vi "Update_Host.vi"(6 "Display Cluster":T1, 7 "ChangeonFly":T2, 8 "SettingsCluster":T3={"Sample Rate (us)"=1, "Samples Per Data Point (int, power of 2)"=1000, "DistanceToBulk (um)"=-1.0, "HoldTimeScaler"=1, "SaveData"=FALSE, "DistanceToBulk (um) 2"=-1.0, "DistanceToBulk (um) 3"=-1.0}, 9 "WayPointCluster":T4) -> ()   [LabVIEW 2023]
uses:
  TypeDefs/WayPointCluster.ctl
  TypeDefs/Settings.ctl
  TypeDefs/ChangeOnFly.ctl
  TypeDefs/Display.ctl
  User_Vi/Settings.vi
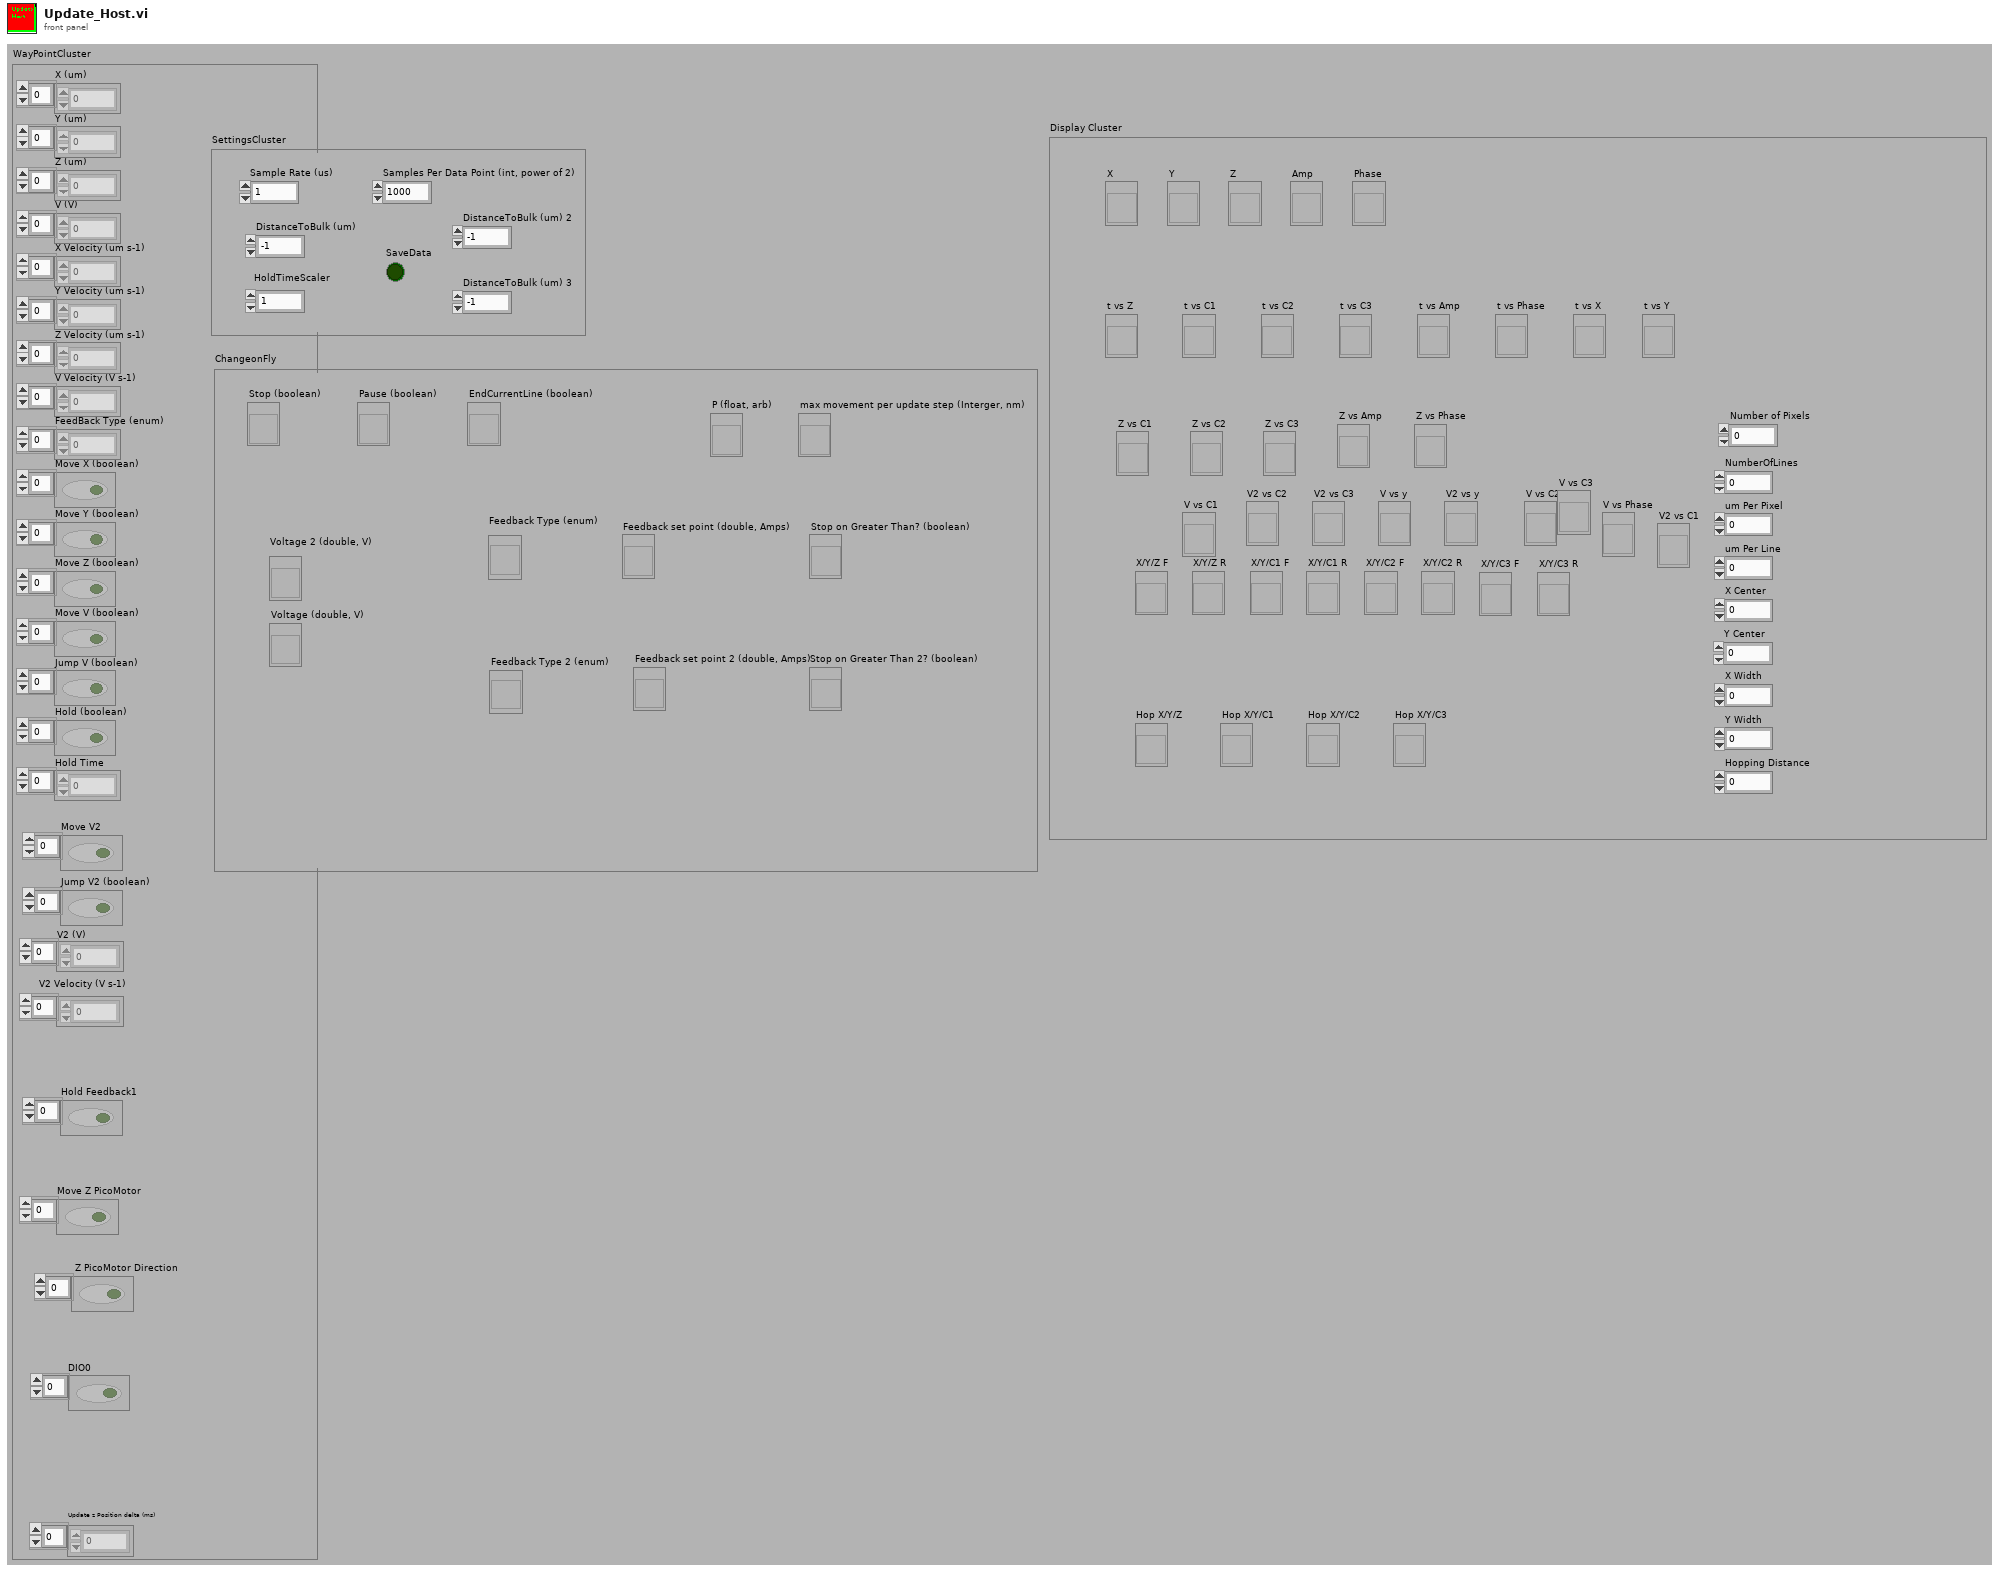
[diagram p1: front panel]
types:
  T1 = typedef "Display.ctl" = cluster{"X":refnum<vi>, "Y":refnum<vi>, "Z":refnum<vi>, "Amp":refnum<vi>, "Phase":refnum<vi>, "t vs Z":refnum<vi>, "t vs C1":refnum<vi>, "t vs C2":refnum<vi>, "t vs C3":refnum<vi>, "t vs Amp":refnum<vi>, "t vs Phase":refnum<vi>, "t vs X":refnum<vi>, "t vs Y":refnum<vi>, "Z vs C1":refnum<vi>, "Z vs C2":refnum<vi>, "Z vs C3":refnum<vi>, "V vs C1":refnum<vi>, "V vs C2":refnum<vi>, "V vs C3":refnum<vi>, "X/Y/Z F":refnum<vi>, "X/Y/Z R":refnum<vi>, "X/Y/C1 F":refnum<vi>, "X/Y/C1 R":refnum<vi>, "X/Y/C2 F":refnum<vi>, "X/Y/C2 R":refnum<vi>, "X/Y/C3 F":refnum<vi>, "X/Y/C3 R":refnum<vi>, "NumberOfLines":u16, "um Per Pixel":dbl, "um Per Line":dbl, "X Center":dbl, "Hop X/Y/Z":refnum<vi>, "Hop X/Y/C1":refnum<vi>, "Hop X/Y/C2":refnum<vi>, "Hop X/Y/C3":refnum<vi>, "X Width":dbl, "Y Width":dbl, "Hopping Distance":dbl, "V2 vs C1":refnum<vi>, "V vs Phase":refnum<vi>, "Y Center":dbl, "Number of Pixels":dbl, "V2 vs C2":refnum<vi>, "V2 vs C3":refnum<vi>, "V vs y":refnum<vi>, "V2 vs y":refnum<vi>, "Z vs Amp":refnum<vi>, "Z vs Phase":refnum<vi>}
  T2 = typedef "ChangeOnFly.ctl" = cluster{"Stop (boolean)":refnum<vi>, "Pause (boolean)":refnum<vi>, "EndCurrentLine (boolean)":refnum<vi>, "max movement per update step (Interger, nm)":refnum<vi>, "P (float, arb)":refnum<vi>, "Feedback set point (double, Amps)":refnum<vi>, "Voltage (double, V)":refnum<vi>, "Feedback set point 2 (double, Amps)":refnum<vi>, "Stop on Greater Than 2? (boolean)":refnum<vi>, "Stop on Greater Than? (boolean)":refnum<vi>, "Voltage 2 (double, V)":refnum<vi>, "Feedback Type (enum)":refnum<vi>, "Feedback Type 2 (enum)":refnum<vi>}
  T3 = typedef "Settings.ctl" = cluster{"Sample Rate (us)":u32, "Samples Per Data Point (int, power of 2)":i16, "DistanceToBulk (um)":dbl, "HoldTimeScaler":u64, "SaveData":bool, "DistanceToBulk (um) 2":dbl, "DistanceToBulk (um) 3":dbl}
  T4 = typedef "WayPointCluster.ctl" = cluster{"X (um)":dbl[], "Y (um)":dbl[], "Z (um)":dbl[], "V (V)":dbl[], "X Velocity (um s-1)":dbl[], "Y Velocity (um s-1)":dbl[], "Z Velocity (um s-1)":dbl[], "V Velocity (V s-1)":dbl[], "FeedBack Type (enum)":u16[], "Move X (boolean)":bool[], "Move Y (boolean)":bool[], "Move Z (boolean)":bool[], "Move V (boolean)":bool[], "Jump V (boolean)":bool[], "Hold (boolean)":bool[], "Hold Time":u32[], "V2 (V)":dbl[], "Move V2":bool[], "V2 Velocity (V s-1)":dbl[], "Jump V2 (boolean)":bool[], "Update z Position delta (ms)":i16[], "Hold Feedback1":bool[], "Move Z PicoMotor":bool[], " Z PicoMotor Direction":bool[], "DIO0":bool[]}
  T5 = enum32{"Bad", "Idle", "Run top level", "Running"}
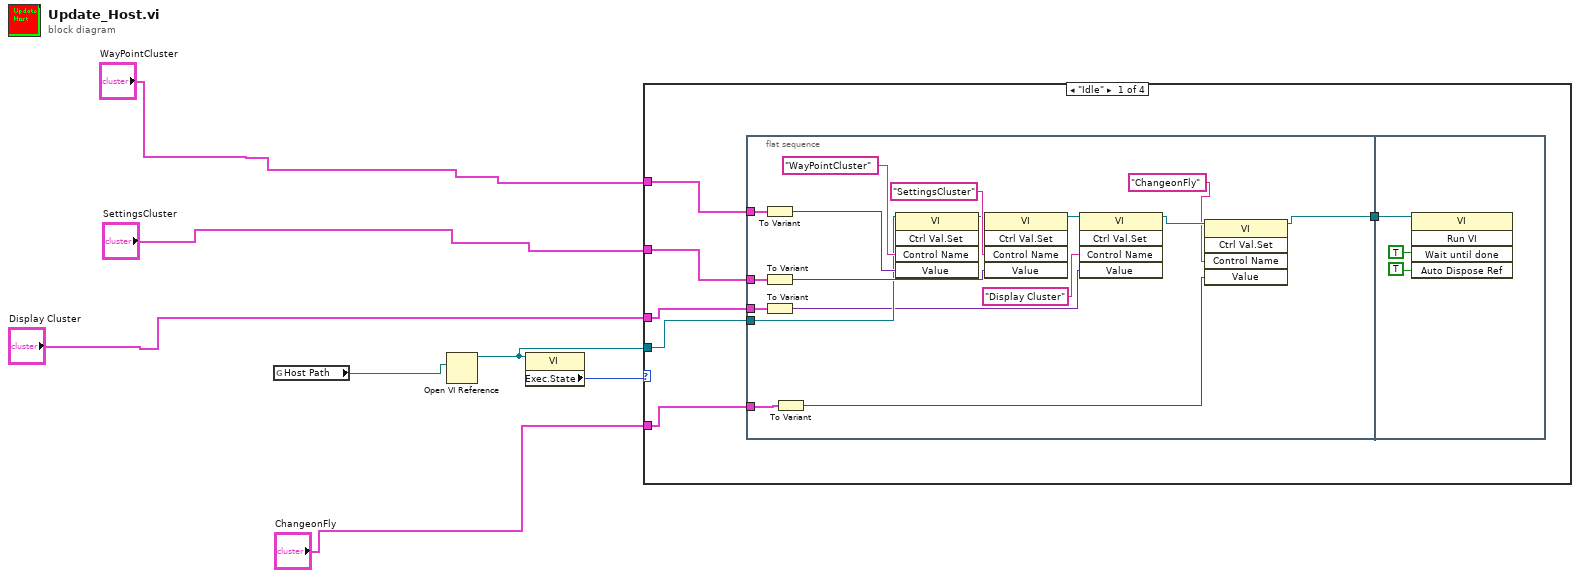
[diagram p0: block diagram]
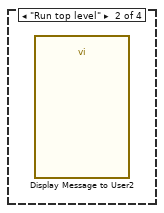
[diagram p2: hidden frame]
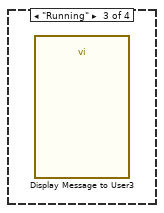
[diagram p3: hidden frame]
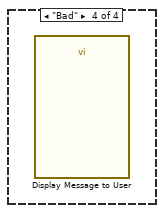
[diagram p4: hidden frame]
diagram:
  n1 = global read "Settings.vi" "Host Path"() -> (w1:path)
  n2 = Open VI Reference(vi path=w1) -> (vi reference=w6:refnum<vi>)  [unwired: 5 in, 1 out]
  n3 = property class="VI"(reference=w6) -> ("Exec.State"=w7:T5)  [unwired: 1 in, 2 out]
  n4 = case shown="\"Idle\"" w7 {
    tunnel: w6 -> [w13 _ _ _]
    tunnel: "WayPointCluster" -> [w12 _ _ _]
    tunnel: "SettingsCluster" -> [w11 _ _ _]
    tunnel: "Display Cluster" -> [w10 _ _ _]
    tunnel: "ChangeonFly" -> [w8 _ _ _]
    frame "Idle" {
      n5 = flat-sequence {
        tunnel: w13 -> [w24]
        tunnel: w12 -> [w29]
        tunnel: w11 -> [w27]
        tunnel: w10 -> [w21]
        tunnel: [w16] -> w9
        tunnel: w8 -> [w18]
        tunnel: w9 -> [w31]
        frame #0 {
          n6 = To Variant(anything=w29) -> (Variant=w28:variant)
          n7 = To Variant(anything=w27) -> (Variant=w26:variant)
          n8 = To Variant(anything=w21) -> (Variant=w20:variant)
          n9 = To Variant(anything=w18) -> (Variant=w14:variant)
          n10 = invoke class="VI" method="Ctrl Val.Set"(reference=w24, "Control Name"="WayPointCluster", "Value"=w28) -> (reference out=w23:refnum<vi>)  [unwired: 2 in, 4 out]
          n11 = invoke class="VI" method="Ctrl Val.Set"(reference=w23, "Control Name"="SettingsCluster", "Value"=w26) -> (reference out=w22:refnum<vi>)  [unwired: 2 in, 4 out]
          n12 = invoke class="VI" method="Ctrl Val.Set"(reference=w22, "Control Name"="Display Cluster", "Value"=w20) -> (reference out=w17:refnum<vi>)  [unwired: 2 in, 4 out]
          n13 = invoke class="VI" method="Ctrl Val.Set"(reference=w17, "Control Name"="ChangeonFly", "Value"=w14) -> (reference out=w16:refnum<vi>)  [unwired: 2 in, 4 out]
        }
        frame #1 {
          n14 = invoke class="VI" method="Run VI"(reference=w31, "Wait until done"=TRUE ("Wait Until Done"), "Auto Dispose Ref"=TRUE ("Auto Dispose Reference")) -> ()  [unwired: 2 in, 5 out]
        }
      }
    }
    frame "Run top level" {
      n15 = call "Display Message to User2"() -> ()  [unwired: 10 in, 2 out]
    }
    frame "Running" {
      n16 = call "Display Message to User3"() -> ()  [unwired: 10 in, 2 out]
    }
    frame "Bad" {
      n17 = call "Display Message to User"() -> ()  [unwired: 10 in, 2 out]
    }
  }
